vi "F to Zmag.vi"(9 "F输入":dbl, 11 "Parameter T1":cluster{"A":dbl, "B":dbl}={"A"=28.06, "B"=-1.501}) -> (2 "Z输出":dbl)   [LabVIEW 2017]
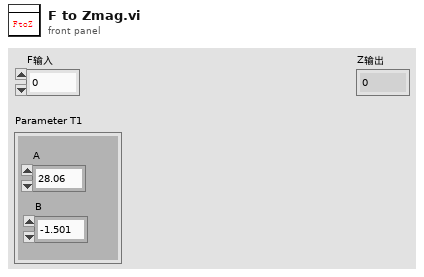
[diagram p1: front panel]
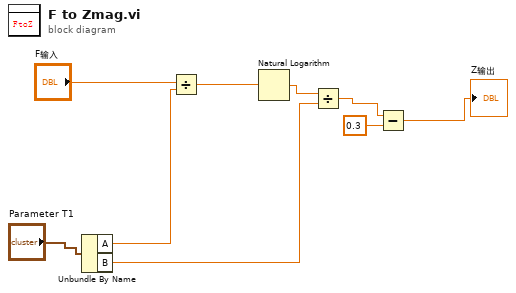
[diagram p0: block diagram]
diagram:
  n1 = Unbundle By Name("Parameter T1") -> ("A"=w5:dbl, "B"=w4:dbl)
  n2 = Divide(x="F输入", y=w5) -> (x/y=w8:dbl)
  n3 = Natural Logarithm(1:w8) -> (0:w9:dbl)
  n4 = Divide(x=w9, y=w4) -> (x/y=w3:dbl)
  n5 = Subtract(x=w3, y=0.3) -> (x-y=→"Z输出":dbl)
